vi "checkFinishPreparePenaltyEnemyPlay.vi"(8 "error in (no error)":errorcluster, 10 "Game":refnum<class "Game.lvclass">, 11 "PreparePenaltyEnemyPlay in":refnum<class "PreparePenaltyEnemyPlay.lvclass">) -> (0 "error out":errorcluster, 2 "Boolean":bool, 3 "PreparePenaltyEnemyPlay out":refnum<class "PreparePenaltyEnemyPlay.lvclass">)   [LabVIEW 2023, in "PreparePenaltyEnemyPlay.lvclass"]
uses:
  PreparePenaltyEnemyPlay.lvclass
  Game_class/Game.lvclass
  Referee_class/command_interpreted.ctl
  Game_class/Game.lvclass/Game.ctl
  Referee_class/Referee.lvclass/Referee.ctl
  Events_class/Events.lvclass/Events.ctl
  Game_class/Read Referee.vi
  Game_class/Read EventsRef.vi
  Events_class/Read ball_out.vi
  Events_class/Read touch.vi
  Events_class/Read id_touch.vi
  Referee_class/Read command_interpreted.vi
  Referee_class/Referee.lvclass
  Events_class/Events.lvclass
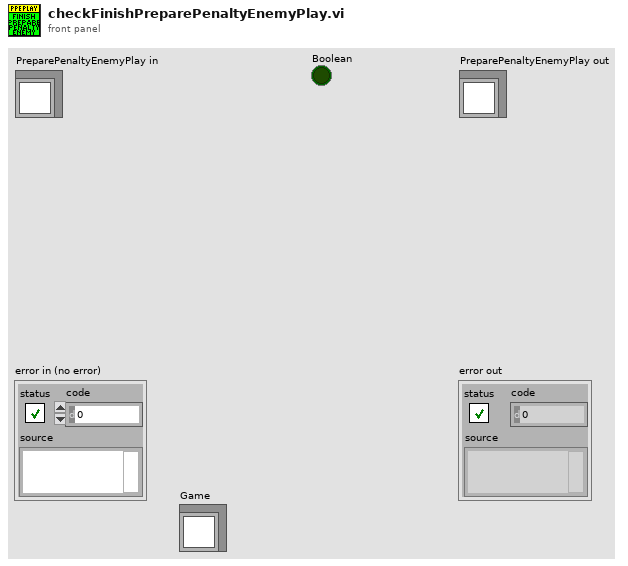
[diagram p1: front panel]
types:
  T1 = typedef "command_interpreted.ctl" = enum16{"Goal Ally", "Goal Enemy", "Ball Placement Enemy", "Ball Placement Ally", "Normal Half Time", "Extra Time  Break", "Extra Half Time", "None", "Post Game", "PKA Normal Start", "Prepare Kickoff Ally", "PKE Normal Start", "Prepare Kickoff Enemy", "Force Start", "Halt", "Timeout", "Prepare Penalty Ally", "Prepare Penalty Enemy", "PPA NormalStart", "PPE Normal Start", "Indirect Free Ally", "Direct Free Enemy", "Direct Free Ally", "Indirect Free Enemy", "Stop"}
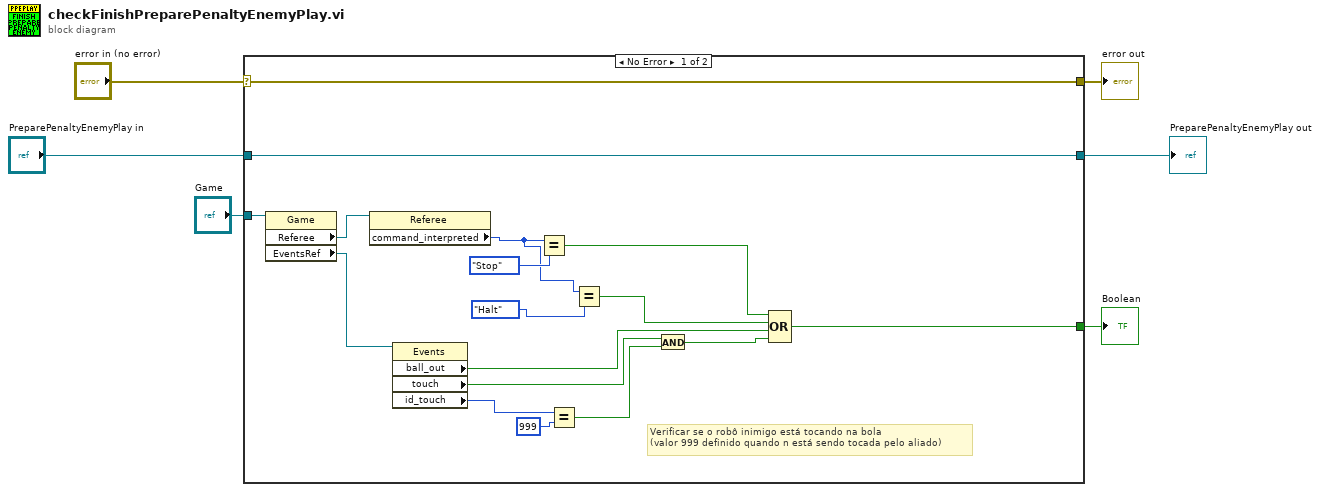
[diagram p0: block diagram]
diagram:
  n1 = case shown="No Error" "error in (no error)" {
    selector: "error in (no error)" -> [w22 w25]
    tunnel: [w22 w25] -> w5
    tunnel: [w23 w24] -> w3
    tunnel: "PreparePenaltyEnemyPlay in" -> [w23 w24]
    tunnel: "Game" -> [w20 _]
    tunnel: [w17 _] -> w1
    frame No Error {
      # "Verificar se o robô inimigo está tocando na bola\n(valor 999 definido quando n está sendo tocada pelo aliado)"
      n2 = property class="Game"(reference=w20) -> ("Referee"=w21:refnum<class "Referee.lvclass">, "EventsRef"=w19:refnum<class "Events.lvclass">)  [unwired: 1 in, 2 out]
      n3 = property class="Referee"(reference=w21) -> ("command_interpreted"=w10:T1)  [unwired: 1 in, 2 out]
      n4 = property class="Events"(reference=w19) -> ("ball_out"=w18:bool, "touch"=w14:bool, "id_touch"=w16:i32)  [unwired: 1 in, 2 out]
      n5 = Equal?(x=w10, y=command_interpreted."Stop") -> (x = y?=w8:bool)
      n6 = Equal?(x=w16, y=999) -> (x = y?=w13:bool)
      n7 = Equal?(x=w10, y=command_interpreted."Halt") -> (x = y?=w7:bool)
      n8 = And(x=w14, y=w13) -> (x .and. y?=w12:bool)
      n9 = Compound Arithmetic op=OR(w8, w7, w18, w12) -> (w17:bool)
    }
    frame Error {
    }
  }
  "error out" <- w5
  "PreparePenaltyEnemyPlay out" <- w3
  "Boolean" <- w1
